vi "LDT Get Message Type.vi"(10 "String":string) -> (2 "submatch 1":string)   [LabVIEW 2022 SP3, in "LDT Telescope.lvclass"]
uses:
  LDT Telescope.lvclass
  <vilib>/regexp/Match Regular Expression.xnode
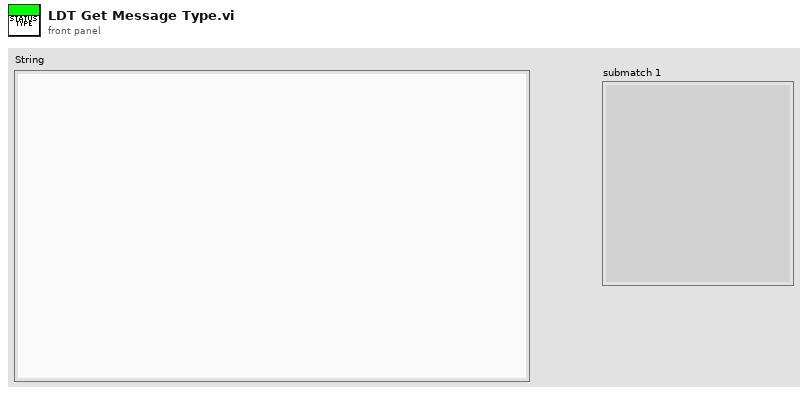
[diagram p1: front panel]
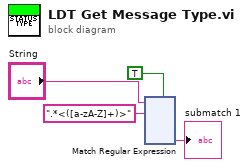
[diagram p0: block diagram]
diagram:
  n1 = xnode "Match Regular Expression"("input string"="String", "regular expression"=".*<([a-zA-Z]+)>", "multiline? (F)"=TRUE) -> ("submatch 1"=→"submatch 1":string)  [unwired: 3 in, 5 out]
